vi "Enumerate Format Names Core.vi"(8 "error in (no error)":errorcluster, 11 "Data Value Reference in":refnum<data-value>) -> (0 "error out":errorcluster, 3 "Map":map{u32, string}(c390))   [LabVIEW 2020, in "g_ar_toolkit.capture.lvlib" / "CameraManager.lvclass"]
uses:
  CameraManager.lvclass
  CameraManager.lvclass/CameraManager.ctl
  bin/g_ar_toolkit.1.32.dll
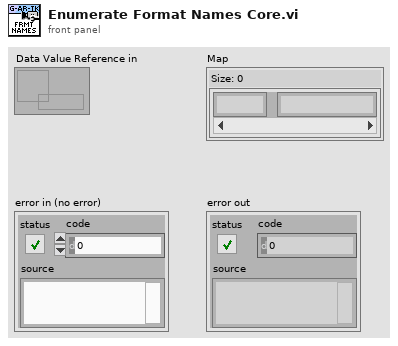
[diagram p1: front panel]
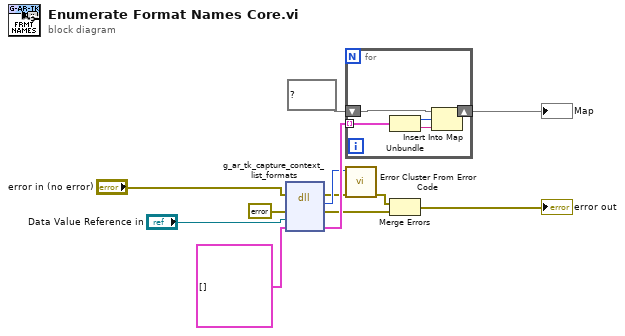
[diagram p0: block diagram]
diagram:
  n1 = dll-call lib="C:/serenial/libraries/g-augmented-reality-toolkit/LabVIEW/bin/g_ar_toolkit.1.*.*" fn="g_ar_tk_capture_context_list_formats" ("g_ar_toolkit.*.*:g_ar_tk_capture_context_enumerate")(error in="error in (no error)", "error_cluster"=errorcluster {"status"=FALSE, "code"=0, "source"=""} ("error constant"), "EDVR"="Data Value Reference in", "device_list"=cluster{"id":u32, "name":string}[] []) -> (error out=w1:errorcluster, "MgErr"=w6:i32, "error_cluster"=w4:errorcluster, "device_list"=w10:cluster{"id":u32, "name":string}[])  [unwired: 3 in, 1 out]
  n2 = for {
    tunnel: w10 -> [w17] mode=indexing
    shift-right: [w14] -> w12
    shift-left: map{u32, string} {} ("Size: 0") -> [w13]
    n3 = Unbundle(w17) -> ("id"=w16:u32, "name"=w15:string)
    n4 = Insert Into Map(map in=w13, key=w16, value=w15) -> (map out=w14:map{u32, string})  [unwired: 2 out]
  }
  "Map" <- w12
  n5 = call <vilib>:"Error Cluster From Error Code.vi"("error in (no error)"=w1, "error code (0)"=w6) -> ("error out"=w2:errorcluster)  [unwired: 7 in]
  n6 = Merge Errors(w2, w4) -> (→"error out":errorcluster)
